vi "Host_AutoApproach_v1.vi"() -> ()   [LabVIEW 2024]
uses:
  <vilib>/FPGAPlugInAG/USB-7845R OEM/niLvFpga_Open_USB-7845R OEM.vi
  <vilib>/rvi/interface/common/dynamic/niFpgaDynamicAddResources.vi
  <vilib>/Utility/error.llb/Error Cluster From Error Code.vi
  <vilib>/rvi/errors/niLvFpgaAdjustHostInterfaceError.vi
  <vilib>/FPGAPlugInAG/Dynamic/niLvFpga_Close_Dynamic.vi
  <vilib>/rvi/interface/nirviOpenFPGA/nirviOpenFPGA.xnode
  FPGA Bitfiles/hoppingsicmv2_FPGATarget_FPGABaselineSamp_R+T2eZOSN-A.lvbitx
  <vilib>/rvi/interface/nirviReadWriteControl/nirviReadWriteControl.xnode
  <vilib>/rvi/interface/nirviCloseFPGA/nirviCloseFPGA.xnode
  FPGA Bitfiles/hoppingsicmv2_FPGATarget_FPGASICMAutoAppr_9u-Tut4ARFs.lvbitx
  <vilib>/rvi/interface/nirviMethod/nirviMethod.xnode
  NiFpgaLv.dll
  <vilib>/rvi/interface/Simulation/niFpgaSimulationCallBeginRW.vi
  <vilib>/rvi/errors/niLvFpgaMergeErrorWithErrorCode.vi
  <vilib>/FPGAPlugInAG/Dynamic/niLvFpga_ReadFifo_Dynamic.vi
  <vilib>/FPGAPlugInAG/Dynamic/niLvFpga_WriteFifo_Dynamic.vi
panel:
  out "Baseline":fxp<+/-,32,16>
  out "ZPiezoPresPos":fxp<+/-,33,17>
  in  "Sensing":enum32{"Feedback Current", "Applied Volts"}(tab)
  out "Current":dbl(graph)
  in  "Positioning":enum32{"Motor + Peizo", "Peizo"}(tab)
  out "OveralPosition":dbl(graph)
  out "PeizoPosition":dbl(graph)
  out "Approached!":bool
  in  "PiezoApproachRate um/s":dbl
  in  "Threshold %":dbl format="%#_13g"
  in  "stop":bool
  out "MotorPosIndex":i32
  # "Default Motor Velocity is 80000"
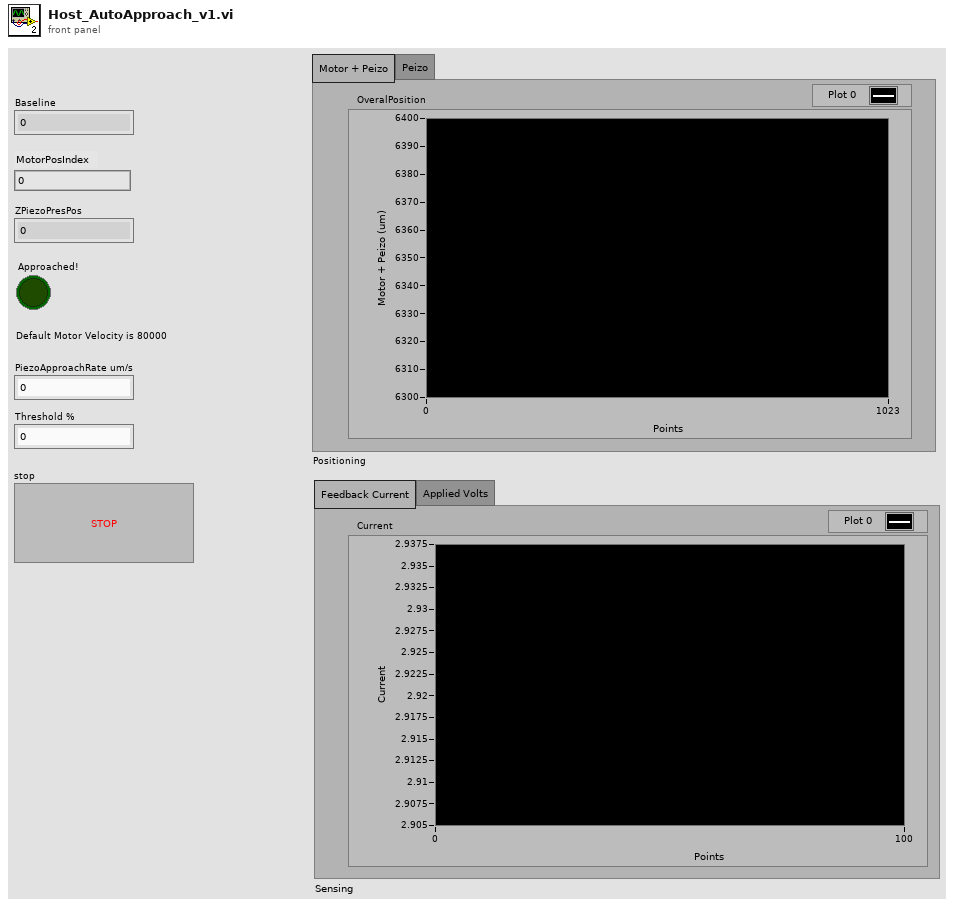
[diagram p1: front panel]
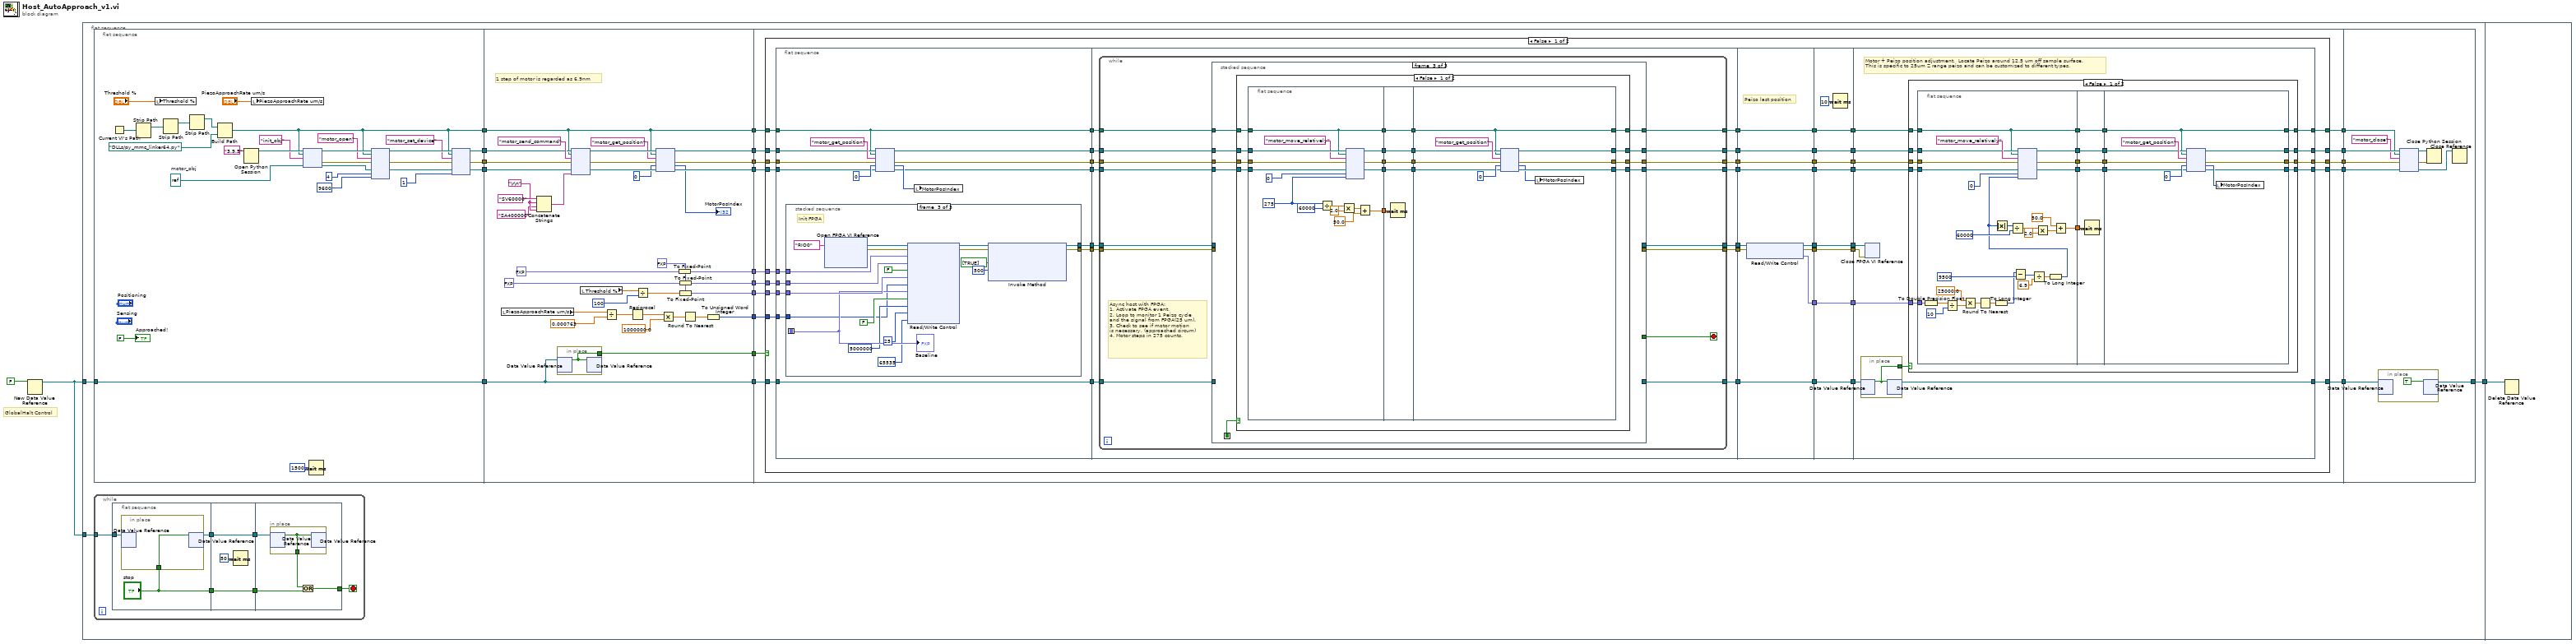
[diagram p0: block diagram]
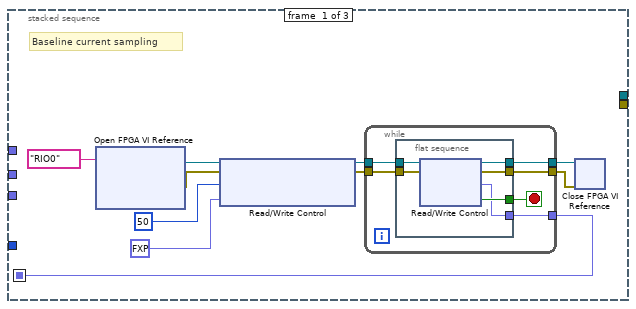
[diagram p2: hidden frame]
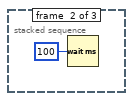
[diagram p3: hidden frame]
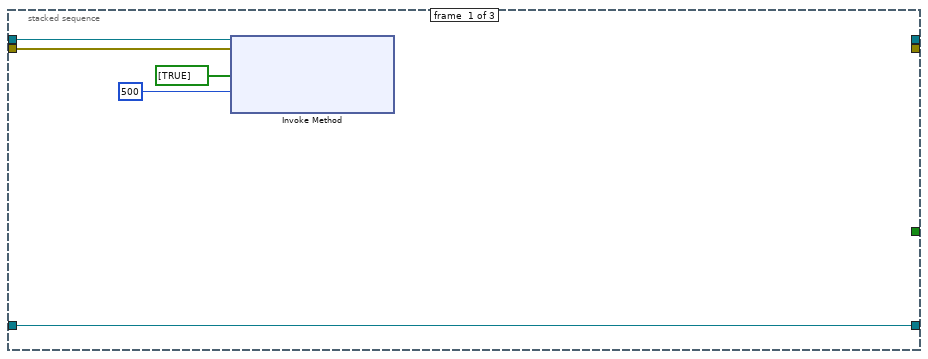
[diagram p4: hidden frame]
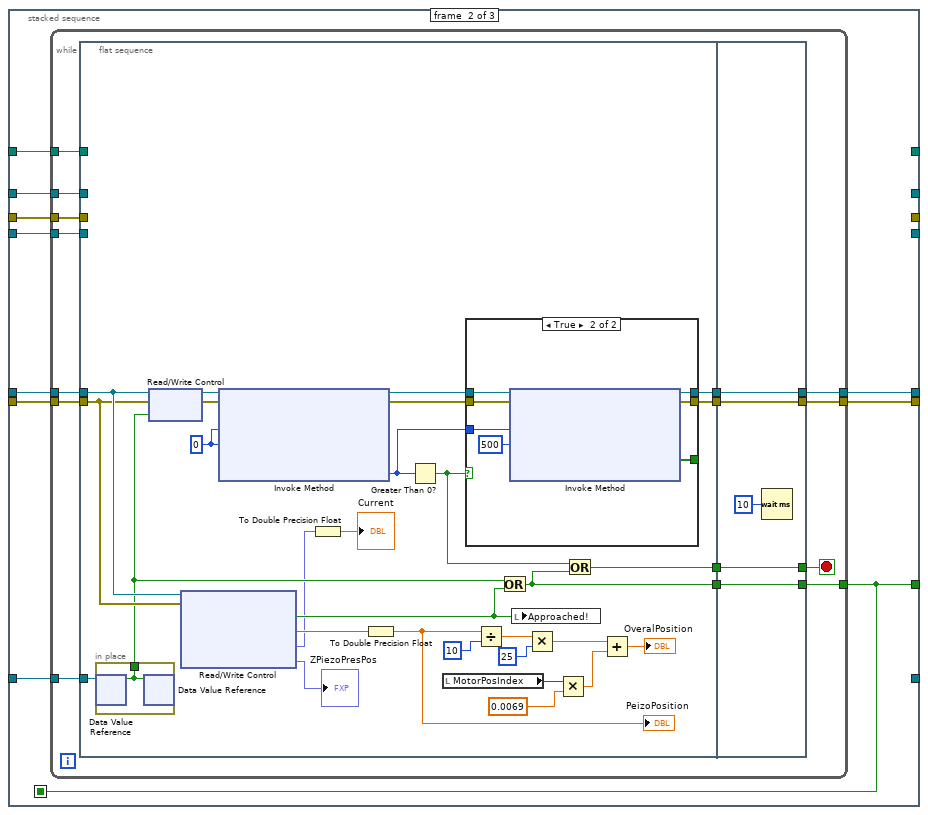
[diagram p5: hidden frame]
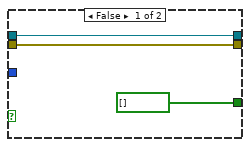
[diagram p6: hidden frame]
diagram:
  # "GlobalHalt Control"
  n1 = New Data Value Reference(data value=FALSE) -> (data value reference=w2:refnum<data-value>)  [unwired: 1 in, 1 out]
  n2 = flat-sequence {
    tunnel: w2 -> [w24]
    tunnel: w2 -> [w23]
    tunnel: [w17] -> w1
    tunnel: w1 -> [w511]
    frame #0 {
      n3 = flat-sequence {
        tunnel: w24 -> [w72]
        tunnel: [w72] -> w26
        tunnel: [w48] -> w15
        tunnel: [w47] -> w14
        tunnel: [w46] -> w13
        tunnel: [w45] -> w12
        tunnel: w26 -> [w110]
        tunnel: [w110] -> w25
        tunnel: [w109] -> w22
        tunnel: [w108] -> w21
        tunnel: [w105] -> w20
        tunnel: [w102] -> w19
        tunnel: [w94] -> w16
        tunnel: w15 -> [w90]
        tunnel: w14 -> [w89]
        tunnel: w13 -> [w88]
        tunnel: w12 -> [w79]
        tunnel: [w79] -> w11
        tunnel: [w78] -> w10
        tunnel: [w77] -> w9
        tunnel: [w76] -> w8
        tunnel: w25 -> [w122]
        tunnel: w22 -> [w126]
        tunnel: w21 -> [w125]
        tunnel: w20 -> [w124]
        tunnel: w19 -> [w123]
        tunnel: [w121] -> w18
        tunnel: w16 -> [w120]
        tunnel: w11 -> [w119]
        tunnel: w10 -> [w118]
        tunnel: w9 -> [w117]
        tunnel: w8 -> [w116]
        tunnel: [w115] -> w7
        tunnel: [w114] -> w6
        tunnel: [w113] -> w5
        tunnel: [w112] -> w4
        tunnel: w18 -> [w509]
        tunnel: [w508] -> w17
        tunnel: w7 -> [w504]
        tunnel: w6 -> [w507]
        tunnel: w5 -> [w506]
        tunnel: w4 -> [w505]
        frame #0 {
          w62 = refnum<k38> refnum  # motor_obj
          n4 = Current VI's Path() -> (path=w66:path)
          n5 = Strip Path(path=w66) -> (stripped path=w65:path)  [unwired: 1 out]
          n6 = local write "Threshold %"("Threshold %") -> ()
          n7 = Strip Path(path=w65) -> (stripped path=w50:path)  [unwired: 1 out]
          n8 = Strip Path(path=w50) -> (stripped path=w49:path)  [unwired: 1 out]
          n9 = Build Path(base path=w49, name or relative path=path "DLLs/py_mmc_linker64.py") -> (appended path=w45:path)
          n10 = Open Python Session(python version="3.9.5" ("Python version")) -> (session out=w67:refnum<k35>)  [unwired: 2 in, 1 out]
          n11 = local write "PiezoApproachRate um/s"("PiezoApproachRate um/s") -> ()
          n12 = node(w67, w45, "init_obj" ("function name"), w62) -> (w61:refnum<k35>, w60:errorcluster, w58:refnum<k38>)  [unwired: 1 in, 2 out]
          n13 = Wait (ms)(milliseconds to wait=u32 1500) -> ()  [unwired: 1 out]
          n14 = node(w61, w45, "motor_open" ("function name"), w60, w58, u8 4 ("COM port select"), 9600 ("COM port select")) -> (w55:refnum<k35>, w54:errorcluster, w53:refnum<k38>)  [unwired: 4 in, 2 out]
          n15 = node(w55, w45, "motor_set_device" ("function name"), w54, w53, u8 1 ("COM port select")) -> (w48:refnum<k35>, w47:errorcluster, w46:refnum<k38>)  [unwired: 3 in, 2 out]
          "Approached!" <- FALSE ("Approached!")
        }
        frame #1 {
          w86 = "\r\n"
          w104 = fxp<+/-,32,16> 0.0 ("fixed-point type")
          # "1 step of motor is regarded as 6.9nm"
          n16 = local read "PiezoApproachRate um/s"() -> (w101:dbl)
          n17 = Concatenate Strings("SV60000", w86, "SA400000", w86) -> (w84:string)
          n18 = in-place {
            in-place-border: [w111] -> w109
            n19 = in-place-dvr #1(w110) -> (w111:bool)  [unwired: 1 out]
            n20 = in-place-dvr #1(w111) -> ()  [unwired: 2 out]
          }
          n21 = node(w90, w79, "motor_send_command" ("function name"), w89, w88, w84) -> (w83:refnum<k35>, w82:errorcluster, w81:refnum<k38>)  [unwired: 3 in, 2 out]
          n22 = local read "Threshold %"() -> (w107:dbl)
          n23 = Divide(x=w101, y=0.000763) -> (x/y=w99:dbl)
          n24 = Reciprocal(x=w99) -> (1/x=w98:dbl)
          n25 = Divide(x=w107, y=100) -> (x/y=w103:dbl)
          n26 = node(w83, w79, "motor_get_position" ("function name"), w82, 0 ("COM port select"), w81) -> (w78:refnum<k35>, w77:errorcluster, →"MotorPosIndex":i32, w76:refnum<k38>)  [unwired: 2 out]
          n27 = Multiply(x=w98, y=1000000.0) -> (x*y=w96:dbl)
          n28 = To Fixed-Point(fixed-point type=w104, number=fxp<+/-,32,8> 4.0 ("PiezoOffsetVolt")) -> (fixed-point=w108:fxp<+/-,32,16>)
          n29 = To Fixed-Point(fixed-point type=w104, number=fxp<+/-,32,8> 6.0 ("PiezoTerminationVolt")) -> (fixed-point=w105:fxp<+/-,32,16>)
          n30 = To Fixed-Point(fixed-point type=w104, number=w103) -> (fixed-point=w102:fxp<+/-,32,16>)
          n31 = Round To Nearest(number=w96) -> (nearest integer value=w95:dbl)
          n32 = To Unsigned Word Integer(number=w95) -> (unsigned 16bit integer=w94:u16)
        }
        frame #2 {
          n33 = case shown="False" w126 {
            tunnel: w125 -> [w168 _]
            tunnel: w124 -> [w167 _]
            tunnel: w123 -> [w166 _]
            tunnel: w122 -> [w165 w499]
            tunnel: [w152 w499] -> w121
            tunnel: w120 -> [w151 _]
            tunnel: w119 -> [w150 w498]
            tunnel: w118 -> [w149 w497]
            tunnel: w117 -> [w148 w496]
            tunnel: w116 -> [w147 w495]
            tunnel: [w130 w498] -> w115
            tunnel: [w129 w497] -> w114
            tunnel: [w128 w496] -> w113
            tunnel: [w127 w495] -> w112
            frame False {
              n34 = flat-sequence {
                tunnel: [w187] -> w170
                tunnel: [w186] -> w169
                tunnel: w168 -> [w185]
                tunnel: w167 -> [w184]
                tunnel: w166 -> [w183]
                tunnel: w165 -> [w182]
                tunnel: [w182] -> w164
                tunnel: w151 -> [w181]
                tunnel: w150 -> [w174]
                tunnel: w149 -> [w178]
                tunnel: w148 -> [w177]
                tunnel: w147 -> [w176]
                tunnel: [w174] -> w146
                tunnel: [w173] -> w145
                tunnel: [w172] -> w144
                tunnel: [w171] -> w143
                tunnel: w170 -> [w243]
                tunnel: w169 -> [w242]
                tunnel: w164 -> [w241]
                tunnel: [w240] -> w163
                tunnel: [w239] -> w162
                tunnel: [w238] -> w161
                tunnel: w146 -> [w237]
                tunnel: w145 -> [w236]
                tunnel: w144 -> [w235]
                tunnel: w143 -> [w234]
                tunnel: [w233] -> w142
                tunnel: [w232] -> w141
                tunnel: [w231] -> w140
                tunnel: [w230] -> w139
                tunnel: [w400] -> w160
                tunnel: [w399] -> w158
                tunnel: [w404] -> w156
                tunnel: [w401] -> w154
                tunnel: w161 -> [w404]
                tunnel: w162 -> [w402]
                tunnel: w163 -> [w403]
                tunnel: w142 -> [w398]
                tunnel: w141 -> [w397]
                tunnel: w140 -> [w396]
                tunnel: w139 -> [w395]
                tunnel: [w398] -> w137
                tunnel: [w397] -> w135
                tunnel: [w396] -> w133
                tunnel: [w395] -> w132
                tunnel: w160 -> [w413]
                tunnel: [w413] -> w159
                tunnel: w158 -> [w412]
                tunnel: [w412] -> w157
                tunnel: w156 -> [w411]
                tunnel: [w411] -> w155
                tunnel: w154 -> [w410]
                tunnel: [w410] -> w153
                tunnel: [w408] -> w138
                tunnel: w137 -> [w408]
                tunnel: [w407] -> w136
                tunnel: w135 -> [w407]
                tunnel: [w406] -> w134
                tunnel: w133 -> [w406]
                tunnel: w132 -> [w405]
                tunnel: [w405] -> w131
                tunnel: w159 -> [w427]
                tunnel: w157 -> [w426]
                tunnel: w155 -> [w425]
                tunnel: w153 -> [w423]
                tunnel: [w422] -> w152
                tunnel: w138 -> [w420]
                tunnel: w136 -> [w421]
                tunnel: w134 -> [w419]
                tunnel: w131 -> [w418]
                tunnel: [w417] -> w130
                tunnel: [w416] -> w129
                tunnel: [w415] -> w128
                tunnel: [w414] -> w127
                frame #0 {
                  n35 = stacked-sequence {
                    seq-local: [w192 _ _] -> [_ _ w225]
                    tunnel: [_ _ w222] -> w187
                    tunnel: [_ _ w221] -> w186
                    tunnel: w185 -> [_ _ w229]
                    tunnel: w184 -> [_ _ w228]
                    tunnel: w183 -> [_ _ w226]
                    tunnel: w181 -> [_ _ w216]
                    frame #0 {
                      # "Baseline current sampling"
                      n36 = xnode "Open FPGA VI Reference"("resource name"=tag "RIO0") -> ("FPGA VI Reference Out"=w190:refnum<k20>, "error out"=w189:errorcluster)  [unwired: 1 in]
                      n37 = xnode "Read/Write Control"("FPGA VI Reference In"=w190, "error in"=w189, "CurrentSampleRate us"=u32 50, "DCVolt V"=fxp<+/-,32,16> 0.0) -> ("FPGA VI Reference Out"=w197:refnum<k20>, "error out"=w196:errorcluster)
                      n38 = while {
                        tunnel: w197 -> [w203]
                        tunnel: w196 -> [w202]
                        tunnel: [w201] -> w195
                        tunnel: [w200] -> w194
                        tunnel: [w198] -> w192
                        stop <- w199 stop-if-true
                        n39 = flat-sequence {
                          tunnel: w203 -> [w209]
                          tunnel: w202 -> [w208]
                          tunnel: [w207] -> w201
                          tunnel: [w206] -> w200
                          tunnel: [w205] -> w199
                          tunnel: [w204] -> w198
                          frame #0 {
                            n40 = xnode "Read/Write Control"("FPGA VI Reference In"=w209, "error in"=w208) -> ("FPGA VI Reference Out"=w207:refnum<k20>, "error out"=w206:errorcluster, "Baseline"=w204:fxp<+/-,32,16>, "Done?"=w205:bool)
                          }
                        }
                      }
                      n41 = xnode "Close FPGA VI Reference"("FPGA VI Reference In"=w195, "error in"=w194) -> ()  [unwired: 1 out]
                    }
                    frame #1 {
                      n42 = Wait (ms)(milliseconds to wait=u32 100) -> ()  [unwired: 1 out]
                    }
                    frame #2 {
                      # "Init FPGA"
                      n43 = xnode "Open FPGA VI Reference"("resource name"=tag "RIO0") -> ("FPGA VI Reference Out"=w214:refnum<k20>, "error out"=w213:errorcluster)  [unwired: 1 in]
                      n44 = xnode "Read/Write Control"("FPGA VI Reference In"=w214, "error in"=w213, "PeizoOffset"=w229, "PeizoMax"=w228, "DeltaMode"=FALSE, "Threshold"=w226, "ApproachRate us"=w216, "BaselineCurrent"=w225, "SurfaceHold"=FALSE, "HoldingElapse us"=u32 5000000, "Retract us/step"=u32 25, "QuietTime us"=u16 65535) -> ("FPGA VI Reference Out"=w224:refnum<k20>, "error out"=w223:errorcluster)
                      n45 = xnode "Invoke Method"("FPGA VI Reference In"=w224, "error in"=w223, "Data"=bool[] [TRUE], "Timeout (ms)"=500) -> ("FPGA VI Reference Out"=w222:refnum<k20>, "error out"=w221:errorcluster)  [unwired: 1 out]
                      "Baseline" <- w225
                    }
                  }
                  n46 = node(w178, w174, "motor_get_position" ("function name"), w177, 0 ("COM port select"), w176) -> (w173:refnum<k35>, w172:errorcluster, w175:i32, w171:refnum<k38>)  [unwired: 2 out]
                  n47 = local write "MotorPosIndex"(w175) -> ()
                }
                frame #1 {
                  n48 = while {
                    tunnel: w243 -> [w258]
                    tunnel: w242 -> [w257]
                    tunnel: w241 -> [w256]
                    tunnel: [w254] -> w240
                    tunnel: [w253] -> w239
                    tunnel: [w252] -> w238
                    tunnel: w237 -> [w251]
                    tunnel: w236 -> [w250]
                    tunnel: w235 -> [w249]
                    tunnel: w234 -> [w248]
                    tunnel: [w247] -> w233
                    tunnel: [w246] -> w232
                    tunnel: [w245] -> w231
                    tunnel: [w244] -> w230
                    stop <- w255 stop-if-true
                    # "Async host with FPGA:\n1. Activate FPGA event.\n2. Loop to monitor 1 Peizo cycle \nand the signal from FPGA(25 um).\n3. Check to see if motor motion \nis necessary. (approached circum) \n4. Motor steps in 275 counts."
                    n49 = stacked-sequence {
                      seq-local: [_ w270 _] -> [_ _ w342]
                      tunnel: w257 -> [w262 w271 _]
                      tunnel: w258 -> [w263 w272 _]
                      tunnel: w256 -> [w260 w273 _]
                      tunnel: [_ w270 _] -> w255
                      tunnel: [_ w269 _] -> w254
                      tunnel: [_ w268 _] -> w253
                      tunnel: [w260 _ _] -> w252
                      tunnel: w251 -> [_ w267 w341]
                      tunnel: w250 -> [_ w266 w340]
                      tunnel: w249 -> [_ w265 w339]
                      tunnel: w248 -> [_ w264 w338]
                      tunnel: [_ _ w337] -> w246
                      tunnel: [_ _ w336] -> w245
                      tunnel: [_ _ w335] -> w244
                      tunnel: [_ _ w334] -> w247
                      frame #0 {
                        n50 = xnode "Invoke Method"("FPGA VI Reference In"=w263, "error in"=w262, "Data"=bool[] [TRUE], "Timeout (ms)"=500) -> ()  [unwired: 3 out]
                      }
                      frame #1 {
                        n51 = while {
                          tunnel: w273 -> [w286]
                          tunnel: w272 -> [w288]
                          tunnel: w271 -> [w287]
                          tunnel: [w283] -> w269
                          tunnel: [w282] -> w268
                          tunnel: [w278] -> w270
                          tunnel: w267 -> [w277]
                          tunnel: w266 -> [w276]
                          tunnel: w265 -> [w275]
                          tunnel: w264 -> [w274]
                          stop <- w280 stop-if-true
                          n52 = flat-sequence {
                            tunnel: w288 -> [w308]
                            tunnel: w287 -> [w307]
                            tunnel: w286 -> [w317]
                            tunnel: [w310] -> w285
                            tunnel: [w309] -> w284
                            tunnel: [w304] -> w281
                            tunnel: [w303] -> w279
                            tunnel: w277 -> [_]
                            tunnel: w276 -> [_]
                            tunnel: w275 -> [_]
                            tunnel: w274 -> [_]
                            tunnel: w285 -> [w332]
                            tunnel: w284 -> [w331]
                            tunnel: [w332] -> w283
                            tunnel: [w331] -> w282
                            tunnel: w281 -> [w330]
                            tunnel: [w330] -> w280
                            tunnel: w279 -> [w329]
                            tunnel: [w329] -> w278
                            frame #0 {
                              w314 = u32 0 ("Number of Elements")
                              n53 = in-place {
                                in-place-border: [w328] -> w306
                                n54 = in-place-dvr #2(w317) -> (w328:bool)  [unwired: 1 out]
                                n55 = in-place-dvr #2(w328) -> ()  [unwired: 2 out]
                              }
                              n56 = xnode "Read/Write Control"("FPGA VI Reference In"=w308, "error in"=w307, "stop"=w306) -> ("FPGA VI Reference Out"=w316:refnum<k20>, "error out"=w315:errorcluster)
                              n57 = xnode "Read/Write Control"("FPGA VI Reference In"=w308, "error in"=w307) -> ("Approached!"=w302:bool, "PeizoFeedbackPos"=w298:fxp<+/-,27,5>, "PresCurr"=w292:fxp<+/-,27,5>, "ZPeizoPresPos"=→"ZPiezoPresPos":fxp<+/-,33,17>)  [unwired: 2 out]
                              n58 = xnode "Invoke Method"("FPGA VI Reference In"=w316, "error in"=w315, "Number of Elements"=w314, "Timeout (ms)"=w314) -> ("FPGA VI Reference Out"=w313:refnum<k20>, "error out"=w312:errorcluster, "Elements Remaining"=w311:u32)  [unwired: 1 out]
                              n59 = To Double Precision Float(number=w292) -> (double precision float=→"Current":dbl)
                              n60 = To Double Precision Float(number=w298) -> (double precision float=w289:dbl)
                              "PeizoPosition" <- w289
                              n61 = Greater Than 0?(x=w311) -> (x > 0?=w305:bool)
                              n62 = local read "MotorPosIndex"() -> (w296:i32)
                              n63 = case shown="True" w305 {
                                tunnel: w313 -> [w320 w327]
                                tunnel: w312 -> [w319 w326]
                                tunnel: w311 -> [_ w325]
                                tunnel: [w320 w323] -> w310
                                tunnel: [w319 w322] -> w309
                                tunnel: [bool[] [] ("Data") w321] -> _
                                frame False {
                                }
                                frame True {
                                n64 = xnode "Invoke Method"("FPGA VI Reference In"=w327, "error in"=w326, "Number of Elements"=w325, "Timeout (ms)"=500) -> ("FPGA VI Reference Out"=w323:refnum<k20>, "error out"=w322:errorcluster, "Data"=w321:bool[])  [unwired: 1 out]
                                }
                              }
                              n65 = Divide(x=w289, y=10) -> (x/y=w300:dbl)
                              n66 = Or(x=w306, y=w302) -> (x .or. y?=w303:bool)
                              n67 = local write "Approached!"(w302) -> ()
                              n68 = Multiply(x=w300, y=25) -> (x*y=w297:dbl)
                              n69 = Multiply(x=w296, y=0.0069) -> (x*y=w294:dbl)
                              n70 = Or(x=w305, y=w303) -> (x .or. y?=w304:bool)
                              n71 = Add(x=w297, y=w294) -> (x+y=→"OveralPosition":dbl)
                            }
                            frame #1 {
                              n72 = Wait (ms)(milliseconds to wait=u32 10) -> ()  [unwired: 1 out]
                            }
                          }
                        }
                      }
                      frame #2 {
                        n73 = case shown="False" w342 {
                          tunnel: w341 -> [w358 w394]
                          tunnel: w340 -> [w357 w393]
                          tunnel: w339 -> [w356 w392]
                          tunnel: w338 -> [w355 w391]
                          tunnel: [w346 w393] -> w337
                          tunnel: [w345 w392] -> w336
                          tunnel: [w344 w391] -> w335
                          tunnel: [w343 w394] -> w334
                          frame False {
                            n74 = flat-sequence {
                              tunnel: [w371] -> w359
                              tunnel: w358 -> [w364]
                              tunnel: w357 -> [w370]
                              tunnel: w356 -> [w369]
                              tunnel: w355 -> [w368]
                              tunnel: [w367] -> w353
                              tunnel: [w366] -> w351
                              tunnel: [w365] -> w349
                              tunnel: [w364] -> w347
                              tunnel: w359 -> [w380]
                              tunnel: [w379] -> w354
                              tunnel: w353 -> [w379]
                              tunnel: [w378] -> w352
                              tunnel: w351 -> [w378]
                              tunnel: [w377] -> w350
                              tunnel: w349 -> [w377]
                              tunnel: [w376] -> w348
                              tunnel: w347 -> [w376]
                              tunnel: w354 -> [w388]
                              tunnel: w352 -> [w387]
                              tunnel: w350 -> [w386]
                              tunnel: w348 -> [w382]
                              tunnel: [w385] -> w346
                              tunnel: [w384] -> w345
                              tunnel: [w383] -> w344
                              tunnel: [w382] -> w343
                              frame #0 {
                                w361 = 275 ("Position Shift [counts]")
                                n75 = Divide(x=w361, y=60000) -> (x/y=w375:dbl)
                                n76 = Multiply(x=w375, y=2.0) -> (x*y=w373:dbl)
                                n77 = node(w370, w364, "motor_move_relatively" ("function name"), w369, w368, 0 ("Axis (0..16)"), w361) -> (w367:refnum<k35>, w366:errorcluster, w365:refnum<k38>)  [unwired: 4 in, 2 out]
                                n78 = Add(x=w373, y=50.0) -> (x+y=w371:dbl)
                              }
                              frame #1 {
                                n79 = Wait (ms)(milliseconds to wait=w380) -> ()  [unwired: 1 out]
                              }
                              frame #2 {
                                n80 = node(w388, w382, "motor_get_position" ("function name"), w387, 0 ("COM port select"), w386) -> (w385:refnum<k35>, w384:errorcluster, w381:i32, w383:refnum<k38>)  [unwired: 2 out]
                                n81 = local write "MotorPosIndex"(w381) -> ()
                              }
                            }
                          }
                          frame True {
                          }
                        }
                      }
                    }
                  }
                }
                frame #2 {
                  # "Peizo last position"
                  n82 = xnode "Read/Write Control"("FPGA VI Reference In"=w403, "error in"=w402) -> ("FPGA VI Reference Out"=w400:refnum<k20>, "error out"=w399:errorcluster, "PeizoThresholdPos"=w401:fxp<+/-,33,17>)
                }
                frame #3 {
                  n83 = Wait (ms)(milliseconds to wait=u32 10) -> ()  [unwired: 1 out]
                }
                frame #4 {
                  # "Motor + Peizo position adjustment.  Locate Peizo around 12.5 um off sample surface. \nThis is specific to 25um Z range peizo and can be customized to different types."
                  n84 = in-place {
                    in-place-border: [w428] -> w424
                    n85 = in-place-dvr #3(w425) -> (w428:bool)  [unwired: 1 out]
                    n86 = in-place-dvr #3(w428) -> (w422:refnum<data-value>)  [unwired: 1 out]
                  }
                  n87 = xnode "Close FPGA VI Reference"("FPGA VI Reference In"=w427, "error in"=w426) -> ()  [unwired: 1 out]
                  n88 = case shown="False" w424 {
                    tunnel: w423 -> [w446 _]
                    tunnel: w421 -> [w444 w493]
                    tunnel: w420 -> [w443 w494]
                    tunnel: w419 -> [w442 w492]
                    tunnel: w418 -> [w441 w491]
                    tunnel: [w432 w494] -> w417
                    tunnel: [w431 w493] -> w416
                    tunnel: [w430 w492] -> w415
                    tunnel: [w429 w491] -> w414
                    frame False {
                      n89 = flat-sequence {
                        tunnel: w446 -> [w475]
                        tunnel: [w460] -> w445
                        tunnel: w444 -> [w454]
                        tunnel: w443 -> [w449]
                        tunnel: w442 -> [w453]
                        tunnel: w441 -> [w452]
                        tunnel: [w450] -> w439
                        tunnel: [w449] -> w437
                        tunnel: [w448] -> w435
                        tunnel: [w447] -> w433
                        tunnel: w445 -> [w480]
                        tunnel: [w479] -> w440
                        tunnel: w439 -> [w479]
                        tunnel: [w478] -> w438
                        tunnel: w437 -> [w478]
                        tunnel: [w477] -> w436
                        tunnel: w435 -> [w477]
                        tunnel: [w476] -> w434
                        tunnel: w433 -> [w476]
                        tunnel: w440 -> [w488]
                        tunnel: w438 -> [w484]
                        tunnel: w436 -> [w487]
                        tunnel: w434 -> [w486]
                        tunnel: [w484] -> w432
                        tunnel: [w483] -> w431
                        tunnel: [w482] -> w430
                        tunnel: [w481] -> w429
                        frame #0 {
                          n90 = To Double Precision Float(number=w475) -> (double precision float=w474:dbl)
                          n91 = Divide(x=w474, y=10) -> (x/y=w472:dbl)
                          n92 = Multiply(x=25000.0, y=w472) -> (x*y=w470:dbl)
                          n93 = Round To Nearest(number=w470) -> (nearest integer value=w469:dbl)
                          n94 = To Long Integer(number=w469) -> (32bit integer=w457:i32)
                          n95 = Subtract(x=w457, y=9500) -> (x-y=w468:i32)
                          n96 = Divide(x=w468, y=6.9 ("x")) -> (x/y=w466:dbl)
                          n97 = To Long Integer(number=w466) -> (32bit integer=w451:i32)
                          n98 = Absolute Value(x=w451) -> (abs(x)=w465:i32)
                          n99 = Divide(x=w465, y=60000) -> (x/y=w464:dbl)
                          n100 = node(w454, w449, "motor_move_relatively" ("function name"), w453, w452, 0 ("Axis (0..16)"), w451) -> (w450:refnum<k35>, w448:errorcluster, w447:refnum<k38>)  [unwired: 4 in, 2 out]
                          n101 = Multiply(x=w464, y=2.0) -> (x*y=w462:dbl)
                          n102 = Add(x=50.0, y=w462) -> (x+y=w460:dbl)
                        }
                        frame #1 {
                          n103 = Wait (ms)(milliseconds to wait=w480) -> ()  [unwired: 1 out]
                        }
                        frame #2 {
                          n104 = node(w488, w484, "motor_get_position" ("function name"), w487, 0 ("COM port select"), w486) -> (w483:refnum<k35>, w482:errorcluster, w485:i32, w481:refnum<k38>)  [unwired: 2 out]
                          n105 = local write "MotorPosIndex"(w485) -> ()
                        }
                      }
                    }
                    frame True {
                    }
                  }
                }
              }
            }
            frame True {
            }
          }
        }
        frame #3 {
          n106 = in-place {
            n107 = in-place-dvr #4(w509) -> ()  [unwired: 2 out]
            n108 = in-place-dvr #4(TRUE ("data value")) -> (w508:refnum<data-value>)  [unwired: 1 out]
          }
          n109 = node(w507, w504, "motor_close" ("function name"), w506, w505) -> (w502:refnum<k35>, w501:errorcluster, w500:refnum<k38>)  [unwired: 2 in, 2 out]
          n110 = Close Python Session(session in=w502, error in=w501) -> ()  [unwired: 1 out]
          n111 = Close Reference(reference=w500) -> ()  [unwired: 1 in, 1 out]
        }
      }
      n112 = while {
        tunnel: w23 -> [w32]
        stop <- w27 stop-if-true
        n113 = flat-sequence {
          tunnel: w32 -> [w35]
          tunnel: ["stop"] -> w30
          tunnel: [w33] -> w28
          tunnel: [w38] -> w31
          tunnel: w30 -> [w38]
          tunnel: [w37] -> w29
          tunnel: w28 -> [w37]
          tunnel: w31 -> [w42]
          tunnel: w29 -> [w43]
          tunnel: [w40] -> w27
          frame #0 {
            n114 = in-place {
              in-place-border: "stop" -> [w36]
              n115 = in-place-dvr #5(w35) -> ()  [unwired: 2 out]
              n116 = in-place-dvr #5(w36) -> (w33:refnum<data-value>)  [unwired: 1 out]
            }
          }
          frame #1 {
            n117 = Wait (ms)(milliseconds to wait=u32 50) -> ()  [unwired: 1 out]
          }
          frame #2 {
            n118 = in-place {
              in-place-border: [w44] -> w41
              n119 = in-place-dvr #6(w43) -> (w44:bool)  [unwired: 1 out]
              n120 = in-place-dvr #6(w44) -> ()  [unwired: 2 out]
            }
            n121 = Or(x=w41, y=w42) -> (x .or. y?=w40:bool)
          }
        }
      }
    }
    frame #1 {
      n122 = Delete Data Value Reference(data value reference=w511) -> ()  [unwired: 1 in, 2 out]
    }
  }
